vi "temporal downsampling.vi"(8 "error in (no error)":errorcluster, 11 "DAQOrcaFlash in":refnum<class "DAQOrcaFlash.lvclass">) -> (0 "error out":errorcluster, 3 "DAQOrcaFlash out":refnum<class "DAQOrcaFlash.lvclass">)   [LabVIEW 2012, in "DAQOrcaFlash.lvclass"]
uses:
  DAQOrcaFlash.lvclass
  dependencies/LabTIFF/LabTIFF/Opening Purpose.ctl
panel:
  out "folder progress":dbl(slide) scale=0.0..1.0
  out "file progress":dbl(slide) scale=0.0..1.0
  in  "cxd folder Path":path
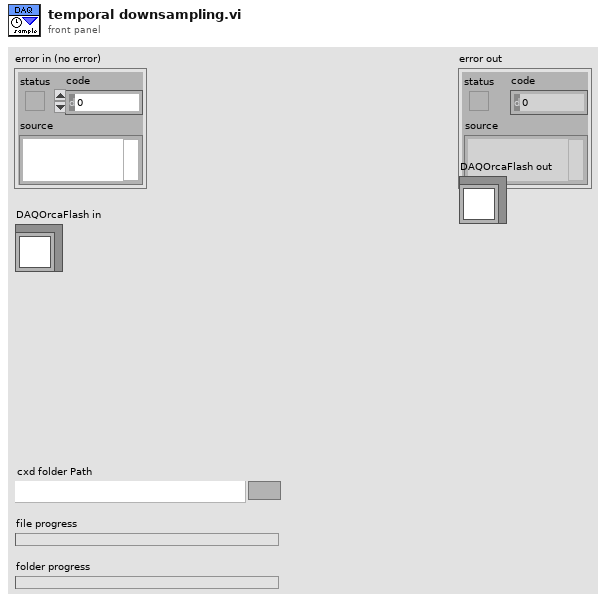
[diagram p1: front panel]
types:
  T1 = typedef "Opening Purpose.ctl" = enum16{"Read", "Write"}
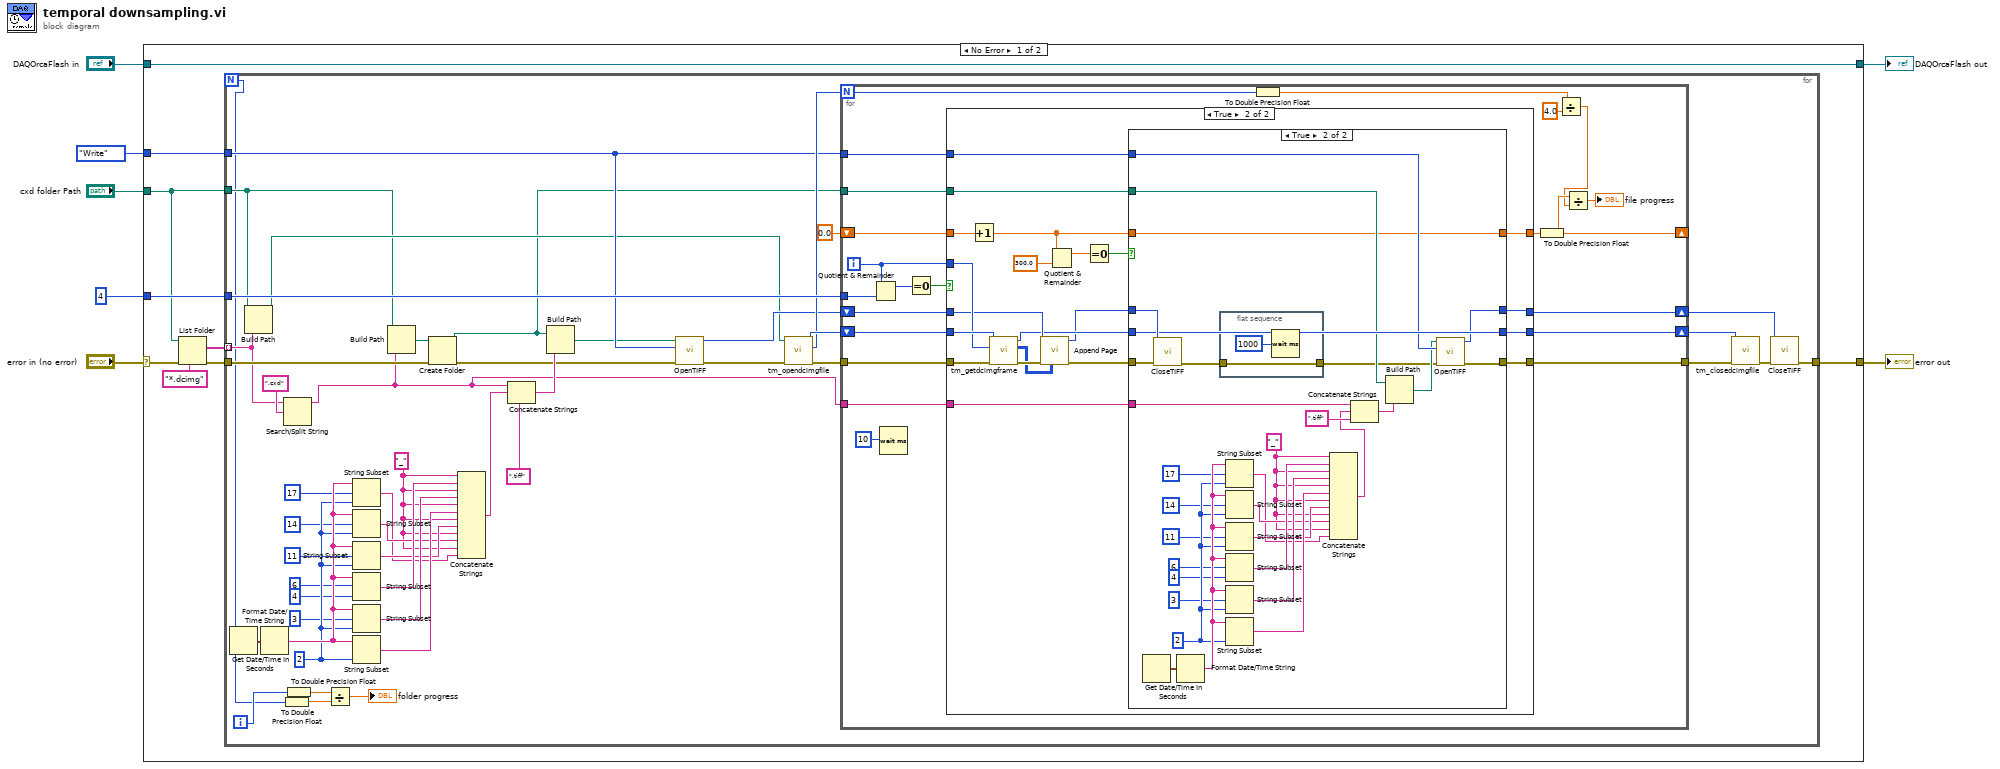
[diagram p0: block diagram]
diagram:
  n1 = case shown="No Error" "error in (no error)" {
    selector: "error in (no error)" -> [w12 w149]
    tunnel: [w14 w149] -> w6
    tunnel: [w16 w148] -> w4
    tunnel: "DAQOrcaFlash in" -> [w16 w148]
    tunnel: Opening_Purpose."Write" ("Opening Purpose") -> [w15 _]
    tunnel: "cxd folder Path" -> [w9 _]
    tunnel: 4 ("temporal downsampling factor") -> [w13 _]
    frame No Error {
      n2 = List Folder(path=w9, pattern="*.dcimg", error in=w12) -> (filenames=w8:string[], error out=w11:errorcluster)  [unwired: 1 in, 2 out]
      n3 = for {
        N -> [w20]
        tunnel: w15 -> [w52]
        tunnel: [w63] -> w14
        tunnel: w13 -> [w62]
        tunnel: w11 -> [w29]
        tunnel: w9 -> [w23]
        tunnel: w8 -> [w27] mode=indexing
        i -> [w21]
        w35 = "_" ("string")
        w48 = 2 ("length (rest)")
        n4 = Get Date/Time In Seconds() -> (seconds since 1Jan1904=w50:timestamp)
        n5 = Build Path(base path=w23, name or relative path=w27) -> (appended path=w26:path)
        n6 = Format Date/Time String(seconds (now)=w50) -> (date/time string=w49:string)  [unwired: 2 in]
        n7 = Search/Split String(string=w27, search string/char (-)=".cxd") -> (substring before match=w24:string)  [unwired: 1 in, 2 out]
        n8 = To Double Precision Float(number=w20) -> (double precision float=w18:dbl)
        n9 = To Double Precision Float(number=w21) -> (double precision float=w19:dbl)
        n10 = Divide(x=w19, y=w18) -> (x/y=→"folder progress":dbl)
        n11 = String Subset(string=w49, offset (0)=17, length (rest)=w48) -> (substring=w36:string)
        n12 = String Subset(string=w49, offset (0)=14, length (rest)=w48) -> (substring=w37:string)
        n13 = String Subset(string=w49, offset (0)=11, length (rest)=w48) -> (substring=w38:string)
        n14 = String Subset(string=w49, offset (0)=6, length (rest)=4 ("length (rest)")) -> (substring=w41:string)
        n15 = String Subset(string=w49, offset (0)=3, length (rest)=w48) -> (substring=w40:string)
        n16 = String Subset(string=w49, length (rest)=w48) -> (substring=w39:string)  [unwired: 1 in]
        n17 = Build Path(base path=w23, name or relative path=w24) -> (appended path=w31:path)
        n18 = Create Folder(path (use dialog)=w31, error in=w29) -> (created path=w22:path, error out=w28:errorcluster)  [unwired: 1 in, 1 out]
        n19 = Concatenate Strings(w35, w41, w35, w40, w35, w39, w35, w38, w35, w37, w35, w36) -> (w33:string)
        n20 = Concatenate Strings(w24, w33, ".tiff" ("string")) -> (w34:string)
        n21 = Build Path(base path=w22, name or relative path=w34) -> (appended path=w30:path)
        n22 = call "OpenTIFF.vi"("error in (no error)"=w28, "Opening Purpose"=w52, "File Path"=w30) -> ("error out"=w58:errorcluster, "TIFF File Ref"=w57:i32)  [unwired: 7 in]
        n23 = call <userlib>:"tm_opendcimgfile.vi"("error in (no error)"=w58, "Path"=w26) -> ("error out"=w60:errorcluster, "Total Frames"=w59:i32, "File Handle"=w61:u32)  [unwired: 7 in]
        n24 = for {
          N: w59 -> [w69]
          tunnel: w60 -> [w84]
          tunnel: [w80] -> w56
          shift-right: [w78] -> w53
          shift-left: w57 -> [w79]
          shift-right: [w77] -> w54
          shift-left: w61 -> [w85]
          tunnel: w62 -> [w76]
          tunnel: w24 -> [w75]
          tunnel: w52 -> [w74]
          tunnel: w22 -> [w73]
          shift-right: [w68] -> _
          shift-left: 0.0 -> [w72]
          i -> [w81]
          n25 = Quotient & Remainder(x=w81, y=w76) -> (x-y*floor(x/y)=w83:i32)  [unwired: 1 out]
          n26 = Wait (ms)(milliseconds to wait=u32 10 ("millisecond timer value")) -> ()  [unwired: 1 out]
          n27 = Equal To 0?(x=w83) -> (x = 0?=w82:bool)
          n28 = case shown="True" w82 {
            tunnel: w85 -> [w87 w110]
            tunnel: w84 -> [w89 w109]
            tunnel: w81 -> [_ w108]
            tunnel: [w89 w104] -> w80
            tunnel: w79 -> [w88 w105]
            tunnel: [w88 w101] -> w78
            tunnel: [w87 w102] -> w77
            tunnel: w75 -> [_ w100]
            tunnel: w74 -> [_ w99]
            tunnel: w73 -> [_ w98]
            tunnel: w72 -> [w86 w95]
            tunnel: [w86 w94] -> w70
            frame False {
            }
            frame True {
              n29 = Increment(x=w95) -> (x+1=w93:dbl)
              n30 = call <userlib>:"tm_getdcimgframe.vi"("error in (no error)"=w109, "Frame Index"=w108, "File Handle in"=w110) -> ("error out"=w107:errorcluster, "Data"=w106:u16[][], "File Handle out"=w103:u32)  [unwired: 5 in, 1 out]
              n31 = call "Append Page.vi"("U16 Image"=w106, "error in (no error)"=w107, "TIFF File Ref"=w105) -> ("error out"=w96:errorcluster, "TIFF File Ref out"=w97:i32)  [unwired: 7 in]
              n32 = Quotient & Remainder(x=w93, y=300.0) -> (x-y*floor(x/y)=w90:dbl)  [unwired: 1 out]
              n33 = Equal To 0?(x=w90) -> (x = 0?=w91:bool)
              n34 = case shown="True" w91 {
                tunnel: w96 -> [w114 w145]
                tunnel: [w114 w136] -> w104
                tunnel: w103 -> [w113 w143]
                tunnel: [w113 w143] -> w102
                tunnel: w97 -> [w112 w144]
                tunnel: [w112 w135] -> w101
                tunnel: w100 -> [_ w115]
                tunnel: w99 -> [_ w142]
                tunnel: w98 -> [_ w141]
                tunnel: w93 -> [w111 w134]
                tunnel: [w111 w134] -> w94
                frame False {
                }
                frame True {
                  w116 = "_" ("string")
                  w132 = 2 ("length (rest)")
                  n35 = Get Date/Time In Seconds() -> (seconds since 1Jan1904=w140:timestamp)
                  n36 = call "CloseTIFF.vi"("error in (no error)"=w145, "TIFF File Ref"=w144) -> ("error out"=w118:errorcluster)  [unwired: 9 in]
                  n37 = Format Date/Time String(seconds (now)=w140) -> (date/time string=w133:string)  [unwired: 2 in]
                  n38 = flat-sequence {
                    tunnel: w118 -> [w146]
                    tunnel: [w146] -> w117
                    frame #0 {
                      n39 = Wait (ms)(milliseconds to wait=u32 1000) -> ()  [unwired: 1 out]
                    }
                  }
                  n40 = String Subset(string=w133, offset (0)=17, length (rest)=w132) -> (substring=w120:string)
                  n41 = String Subset(string=w133, offset (0)=14, length (rest)=w132) -> (substring=w121:string)
                  n42 = String Subset(string=w133, offset (0)=11, length (rest)=w132) -> (substring=w122:string)
                  n43 = String Subset(string=w133, offset (0)=6, length (rest)=4 ("length (rest)")) -> (substring=w125:string)
                  n44 = String Subset(string=w133, offset (0)=3, length (rest)=w132) -> (substring=w124:string)
                  n45 = String Subset(string=w133, length (rest)=w132) -> (substring=w123:string)  [unwired: 1 in]
                  n46 = Concatenate Strings(w116, w125, w116, w124, w116, w123, w116, w122, w116, w121, w116, w120) -> (w119:string)
                  n47 = Concatenate Strings(w115, w119, ".tiff" ("search string/char (-)")) -> (w138:string)
                  n48 = Build Path(base path=w141, name or relative path=w138) -> (appended path=w137:path)
                  n49 = call "OpenTIFF.vi"("error in (no error)"=w117, "Opening Purpose"=w142, "File Path"=w137) -> ("error out"=w136:errorcluster, "TIFF File Ref"=w135:i32)  [unwired: 7 in]
                }
              }
            }
          }
          n50 = To Double Precision Float(number=w69) -> (double precision float=w65:dbl)
          n51 = To Double Precision Float(number=w70) -> (double precision float=w68:dbl)
          n52 = Divide(x=w65, y=4.0) -> (x/y=w64:dbl)
          n53 = Divide(x=w68, y=w64) -> (x/y=→"file progress":dbl)
        }
        n54 = call <userlib>:"tm_closedcimgfile.vi"("error in (no error)"=w56, "File Handle"=w54) -> ("error out"=w55:errorcluster)  [unwired: 9 in]
        n55 = call "CloseTIFF.vi"("error in (no error)"=w55, "TIFF File Ref"=w53) -> ("error out"=w63:errorcluster)  [unwired: 9 in]
      }
    }
    frame Error {
    }
  }
  "error out" <- w6
  "DAQOrcaFlash out" <- w4
